vi "RPC Server Template.vi"(8 "error in (no error)":errorcluster) -> (0 "error out":errorcluster)   [LabVIEW 2015, in "JSONRPC Server.lvclass"]
doc: "Use this as a starting point for the RPC Server processing loop in your application"
uses:
  JSONRPC Server.lvclass
  Request/Request.lvclass/Request.ctl
  Request/Read method.vi
  Request/Read params.vi
  <vilib>/NI/i3 JSON/JSON Generation/Create Value Files/Create Value - String.vi
  Add Response (Method Not Found from Request).vi
  <vilib>/NI/i3 JSON/JSON Parsing/Get Array Value at Index Files/Get Array Value at Index - Numeric.vi
  <vilib>/NI/i3 JSON/JSON Generation/Create Value Files/Create Value - Numeric.vi
  Add Response (Result from Request).vi
  Add Response (Invalid Params from Request).vi
  Add Response (Server Error from Request).vi
  params/params.lvclass
  <vilib>/NI/i3 JSON/i3-json.lvlib
  Request/Request.lvclass
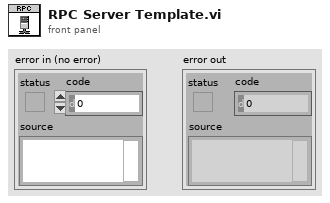
[diagram p1: front panel]
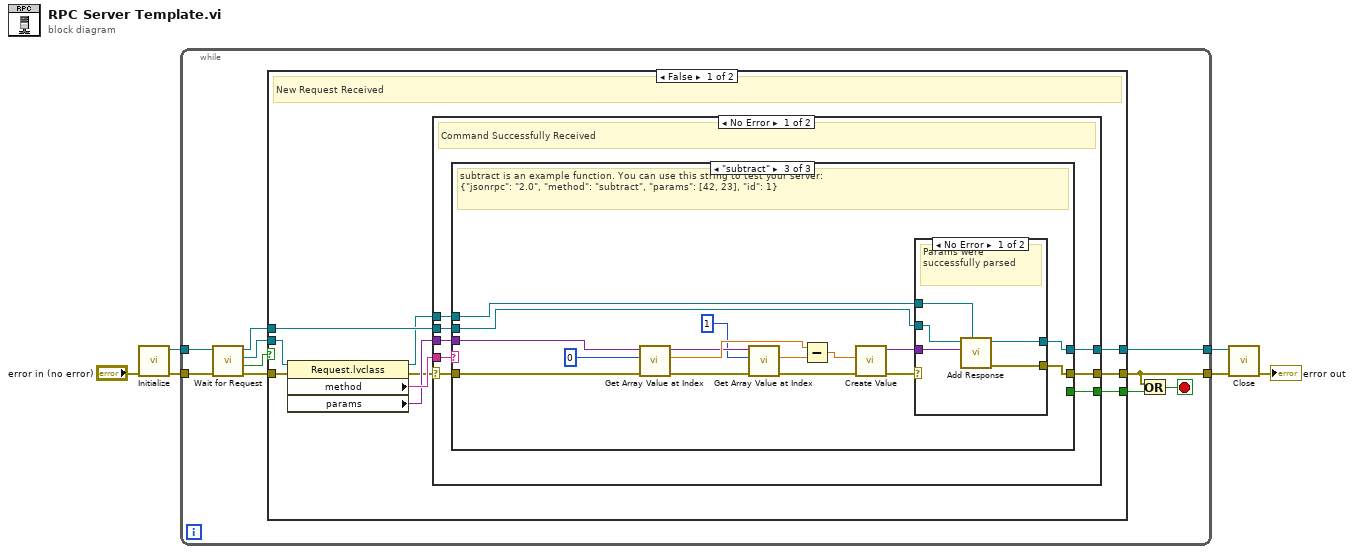
[diagram p0: block diagram]
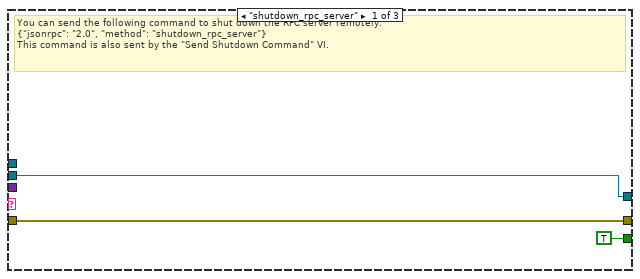
[diagram p2: hidden frame]
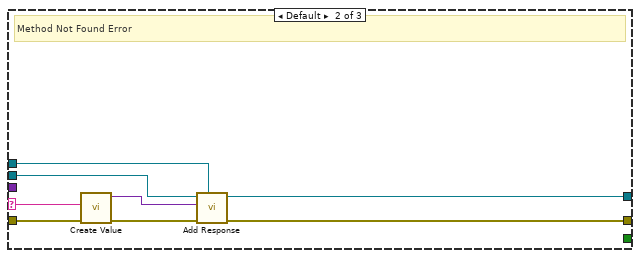
[diagram p3: hidden frame]
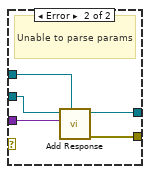
[diagram p4: hidden frame]
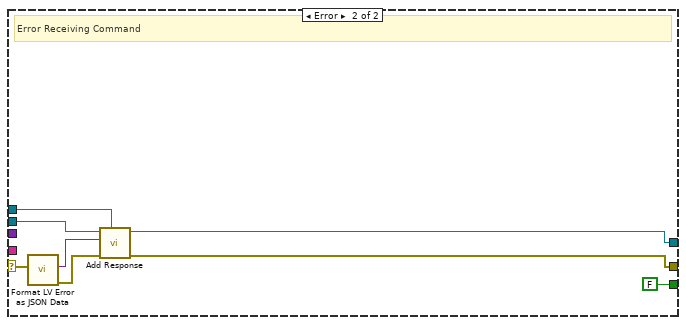
[diagram p5: hidden frame]
diagram:
  n1 = call "Initialize.vi"("error in (no error)"="error in (no error)") -> ("error out"=w5:errorcluster, "Server Out"=w6:refnum<class "JSONRPC Server.lvclass">)  [unwired: 9 in]
  n2 = while {
    tunnel: w6 -> [w16]
    tunnel: w5 -> [w12]
    tunnel: [w8] -> w3
    tunnel: [w10] -> w4
    stop <- w7 stop-if-true
    n3 = call "Wait for Request.vi"("error in (no error)"=w12, "Server in"=w16) -> ("error out"=w11:errorcluster, "timed out?"=w13:bool, "element"=w14:refnum<class "Request.lvclass">, "Server out"=w15:refnum<class "JSONRPC Server.lvclass">)  [unwired: 6 in]
    n4 = case shown="False" w13 {
      tunnel: w15 -> [w19 w80]
      tunnel: w14 -> [w26 _]
      tunnel: w11 -> [w23 w81]
      tunnel: [w21 w81] -> w8
      tunnel: [w20 _] -> w9
      tunnel: [w18 w80] -> w10
      frame False {
        # "New Request Received"
        n5 = property class="Request.lvclass"(reference=w26, error in=w23) -> (reference out=w17:refnum<class "Request.lvclass">, error out=w22:errorcluster, "method"=w25:string, "params"=w24:variant)
        n6 = case shown="No Error" w22 {
          selector: w22 -> [w32 w73]
          tunnel: w25 -> [w34 _]
          tunnel: w24 -> [w33 _]
          tunnel: [w31 w76] -> w21
          tunnel: [w30 FALSE] -> w20
          tunnel: w19 -> [w29 w78]
          tunnel: [w28 w77] -> w18
          tunnel: w17 -> [w27 w79]
          frame No Error {
            # "Command Successfully Received"
            n7 = case shown="\"subtract\"" w34 {
              selector: w34 -> [_ w43 _]
              tunnel: w33 -> [_ _ w58]
              tunnel: w32 -> [w36 w39 w56]
              tunnel: [w36 w41 w48] -> w31
              tunnel: [TRUE _ _] -> w30
              tunnel: w29 -> [w35 w45 w51]
              tunnel: [w35 w40 w50] -> w28
              tunnel: w27 -> [_ w44 w47]
              frame "shutdown_rpc_server" {
                # "You can send the following command to shut down the RPC server remotely:\n{\"jsonrpc\": \"2.0\", \"method\": \"shutdown_rpc_server\"}\nThis command is also sent by the \"Send Shutdown Command\" VI."
              }
              frame Default {
                # "Method Not Found Error"
                n8 = call-poly <vilib>:"Create Value.vi"("error in (no error)"=w39, "String"=w43) -> ("error out"=w38:errorcluster, "JSON Tree"=w42:variant)  [unwired: 8 in]
                n9 = call-poly "Add Response.vi"("Request"=w44, "error in (no error)"=w38, "data"=w42, "Server in"=w45) -> ("error out"=w41:errorcluster, "Server out"=w40:refnum<class "JSONRPC Server.lvclass">)  [unwired: 6 in]
              }
              frame "subtract" {
                # "subtract is an example function. You can use this string to test your server:\n{\"jsonrpc\": \"2.0\", \"method\": \"subtract\", \"params\": [42, 23], \"id\": 1}"
                n10 = call-poly <vilib>:"Get Array Value at Index.vi"("error in (no error)"=w56, "Index"=0, "JSON Tree In (JSON Array)"=w58) -> ("error out"=w55:errorcluster, "Double Value"=w60:dbl, "JSON Tree Out Passthrough"=w57:variant)  [unwired: 5 in, 1 out]
                n11 = call-poly <vilib>:"Get Array Value at Index.vi"("error in (no error)"=w55, "Index"=1, "JSON Tree In (JSON Array)"=w57) -> ("error out"=w54:errorcluster, "Double Value"=w59:dbl)  [unwired: 5 in, 2 out]
                n12 = Subtract(x=w60, y=w59) -> (x-y=w61:dbl)
                n13 = call-poly <vilib>:"Create Value.vi"("error in (no error)"=w54, "Numeric"=w61) -> ("error out"=w46:errorcluster, "JSON Tree"=w49:variant)  [unwired: 8 in]
                n14 = case shown="No Error" w46 {
                  tunnel: w51 -> [w66 w71]
                  tunnel: [w65 w70] -> w50
                  tunnel: w49 -> [w64 w69]
                  tunnel: [w63 w68] -> w48
                  tunnel: w47 -> [w62 w67]
                  frame No Error {
                    # "Params were successfully parsed"
                    n15 = call-poly "Add Response.vi"("Request"=w62, "Response JSON Tree In"=w64, "Server in"=w66) -> ("error out"=w63:errorcluster, "Server out"=w65:refnum<class "JSONRPC Server.lvclass">)  [unwired: 7 in]
                  }
                  frame Error {
                    # "Unable to parse params"
                    n16 = call-poly "Add Response.vi"("Request"=w67, "data"=w69, "Server in"=w71) -> ("error out"=w68:errorcluster, "Server out"=w70:refnum<class "JSONRPC Server.lvclass">)  [unwired: 7 in]
                  }
                }
              }
            }
          }
          frame Error {
            # "Error Receiving Command"
            n17 = call "Format LV Error as JSON Data.vi"("error in"=w73) -> ("error out"=w74:errorcluster, "Error Data Out"=w72:variant)  [unwired: 9 in]
            n18 = call-poly "Add Response.vi"("Request"=w79, "error in (no error)"=w74, "data"=w72, "Server in"=w78) -> ("error out"=w76:errorcluster, "Server out"=w77:refnum<class "JSONRPC Server.lvclass">)  [unwired: 6 in]
          }
        }
      }
      frame True {
        # "Timeout while waiting for new Requests"
      }
    }
    n19 = Or(x=w8, y=w9) -> (x .or. y?=w7:bool)
  }
  n20 = call-dynamic "Close.vi"("error in (no error)"=w3, "Server in"=w4) -> ("error out"=→"error out":errorcluster)  [unwired: 9 in]
